vi "McPherson Set X V.vi"(0 "VISA Resource Name":refnum<visa-resource-name>, 1 "milliseconds to wait":u32=10, 2 "SetValue In":i32, 3 "error In":errorcluster, 4 "Action":enum16{"Stop", "MoveTo", "SpeedAt"}(ring)) -> (5 "dup VISA Resource Name":refnum<visa-resource-name>, 6 "SetValue Out":i32, 7 "error out":errorcluster)   [LabVIEW 2020]
uses:
  Serial Instruments/Serial Support VISA.llb/Serial Actions.ctl
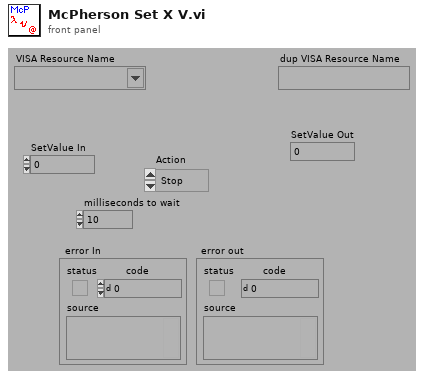
[diagram p1: front panel]
types:
  T1 = typedef "Serial Actions.ctl" = enum16{"Init", "Break", "Clear Buffer", "Write", "Read", "N Bytes", "Lock", "Unlock", "Close"}
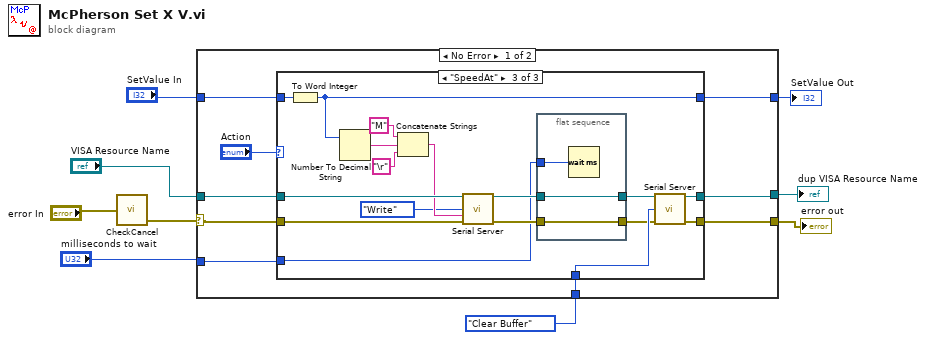
[diagram p0: block diagram]
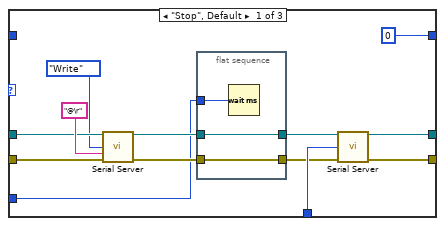
[diagram p2: hidden frame]
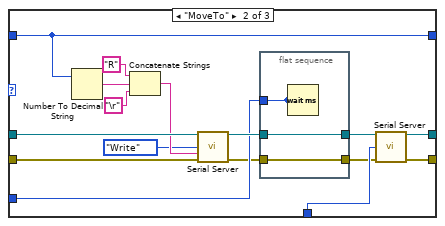
[diagram p3: hidden frame]
diagram:
  n1 = call "CheckCancel.vi"("error in (no error)"="error In") -> ("error out"=w5:errorcluster)  [unwired: 1 in, 1 out]
  n2 = case shown="No Error" w5 {
    selector: w5 -> [w14 w74]
    tunnel: "VISA Resource Name" -> [w18 w75]
    tunnel: "milliseconds to wait" -> [w16 _]
    tunnel: Serial_Actions."Clear Buffer" ("Action") -> [w15 _]
    tunnel: [w13 w74] -> w4
    tunnel: [w12 w75] -> w3
    tunnel: [w11 w76] -> w2
    tunnel: "SetValue In" -> [w10 w76]
    frame No Error {
      n3 = case "Case" shown="\"SpeedAt\"" "Action" {
        tunnel: [w27 w46 w65] -> w13
        tunnel: w14 -> [w30 w43 w62]
        tunnel: w18 -> [w29 w42 w61]
        tunnel: [0 ("SetValue In") w47 w67] -> w11
        tunnel: w10 -> [_ w47 w66]
        tunnel: [w26 w45 w64] -> w12
        tunnel: w16 -> [w20 w36 w54]
        tunnel: w15 -> [w28 w44 w63]
        frame "Stop", Default {
          n4 = call "Serial Server.vi"("VISA Resource Name"=w29, "Action"=Serial_Actions."Write", "String To Send"="@\r" ("Substring"), "error in (no error)"=w30) -> ("dup VISA Resource Name"=w23:refnum<visa-resource-name>, "error out"=w24:errorcluster)  [unwired: 7 in, 3 out]
          n5 = flat-sequence {
            tunnel: [w34] -> w21
            tunnel: w24 -> [w34]
            tunnel: [w33] -> w22
            tunnel: w23 -> [w33]
            tunnel: w20 -> [w32]
            frame #0 {
              n6 = Wait (ms)(milliseconds to wait=w32) -> ()  [unwired: 1 out]
            }
          }
          n7 = call "Serial Server.vi"("VISA Resource Name"=w22, "Action"=w28, "error in (no error)"=w21) -> ("dup VISA Resource Name"=w26:refnum<visa-resource-name>, "error out"=w27:errorcluster)  [unwired: 8 in, 3 out]
        }
        frame "MoveTo" {
          n8 = Number To Decimal String(number=w47) -> (decimal integer string=w49:string)  [unwired: 1 in]
          n9 = Concatenate Strings("R" ("Substring"), w49, "\r" ("Substring")) -> (w41:string)
          n10 = call "Serial Server.vi"("VISA Resource Name"=w42, "Action"=Serial_Actions."Write", "String To Send"=w41, "error in (no error)"=w43) -> ("dup VISA Resource Name"=w38:refnum<visa-resource-name>, "error out"=w35:errorcluster)  [unwired: 7 in, 3 out]
          n11 = flat-sequence {
            tunnel: [w53] -> w39
            tunnel: w35 -> [w53]
            tunnel: [w52] -> w37
            tunnel: w38 -> [w52]
            tunnel: [w51] -> _
            tunnel: w36 -> [w51]
            frame #0 {
              n12 = Wait (ms)(milliseconds to wait=w51) -> ()  [unwired: 1 out]
            }
          }
          n13 = call "Serial Server.vi"("VISA Resource Name"=w37, "Action"=w44, "error in (no error)"=w39) -> ("dup VISA Resource Name"=w45:refnum<visa-resource-name>, "error out"=w46:errorcluster)  [unwired: 8 in, 3 out]
        }
        frame "SpeedAt" {
          n14 = To Word Integer(number=w66) -> (16bit integer=w67:i16)
          n15 = Number To Decimal String(number=w67) -> (decimal integer string=w69:string)  [unwired: 1 in]
          n16 = Concatenate Strings("M" ("Substring"), w69, "\r" ("Substring")) -> (w60:string)
          n17 = call "Serial Server.vi"("VISA Resource Name"=w61, "Action"=Serial_Actions."Write", "String To Send"=w60, "error in (no error)"=w62) -> ("dup VISA Resource Name"=w56:refnum<visa-resource-name>, "error out"=w58:errorcluster)  [unwired: 7 in, 3 out]
          n18 = flat-sequence {
            tunnel: [w73] -> w57
            tunnel: w58 -> [w73]
            tunnel: [w72] -> w55
            tunnel: w56 -> [w72]
            tunnel: w54 -> [w71]
            frame #0 {
              n19 = Wait (ms)(milliseconds to wait=w71) -> ()  [unwired: 1 out]
            }
          }
          n20 = call "Serial Server.vi"("VISA Resource Name"=w55, "Action"=w63, "error in (no error)"=w57) -> ("dup VISA Resource Name"=w64:refnum<visa-resource-name>, "error out"=w65:errorcluster)  [unwired: 8 in, 3 out]
        }
      }
    }
    frame Error {
    }
  }
  "dup VISA Resource Name" <- w3
  "error out" <- w4
  "SetValue Out" <- w2
